vi "Glove box startup.vi"() -> ()   [LabVIEW 2017]
uses:
  <instrlib>/SST sensing O2 sensor/SST sensing O2 sensor.lvlib
panel:
  out "O2 free reached":bool
  in  "Off threshold %":dbl=1.0
  out "O2 level %":dbl
  out "O2 level Chart":dbl(graph)
  in  "Start N2 purge":bool
  in  "stop":bool
  out "Sensor status":string="Idle"
  in  "O2 sensor On/Off":bool
  in  "O2 sensor COM":refnum<visa-resource-name>="COM18"
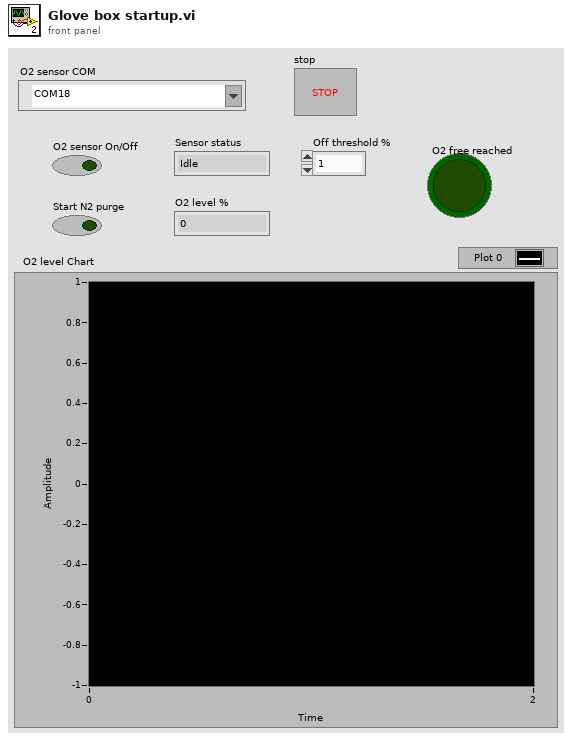
[diagram p1: front panel]
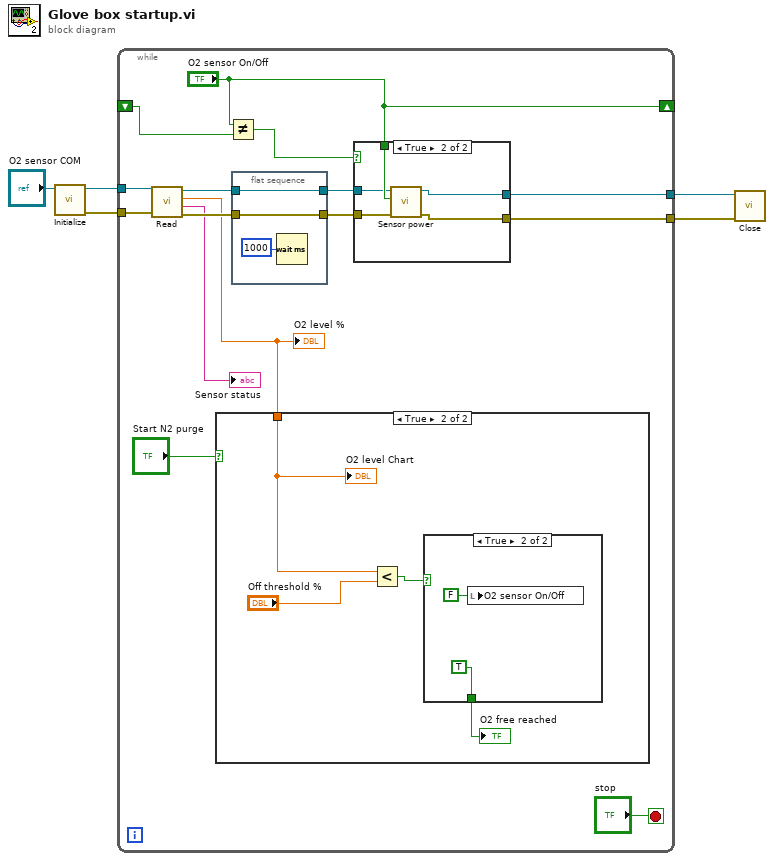
[diagram p0: block diagram]
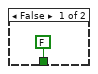
[diagram p3: hidden frame]
diagram:
  n1 = call <instrlib>:"Initialize.vi"("COM port"="O2 sensor COM") -> ("error out"=w3:errorcluster, "Modbus instance"=w4:refnum<class "Modbus Master.lvclass">)  [unwired: 9 in]
  n2 = while {
    tunnel: w4 -> [w20]
    tunnel: w3 -> [w19]
    shift-right: ["O2 sensor On/Off"] -> _
    shift-left: _ -> [w17]
    tunnel: [w10] -> w2
    tunnel: [w9] -> w1
    stop <- "stop" stop-if-true
    n3 = call <instrlib>:"Read.vi"("error in (no error)"=w19, "Modbus master in"=w20) -> ("error out"=w12:errorcluster, "Status"=→"Sensor status":string, "O2 level %"=w6:dbl, "Modbus master out"=w14:refnum<class "Modbus Master.lvclass">)  [unwired: 6 in]
    "O2 level %" <- w6
    n4 = case shown="True" "Start N2 purge" {
      tunnel: w6 -> [_ w24]
      frame False {
      }
      frame True {
        n5 = Less?(x=w24, y="Off threshold %") -> (x < y?=w22:bool)
        n6 = case shown="True" w22 {
          tunnel: [FALSE ("O2 free reached") TRUE ("O2 free reached")] -> w21
          frame False {
          }
          frame True {
            n7 = local write "O2 sensor On/Off"(FALSE ("O2 sensor On/Off")) -> ()
          }
        }
        "O2 free reached" <- w21
        "O2 level Chart" <- w24
      }
    }
    n8 = Not Equal?(x="O2 sensor On/Off", y=w17) -> (x != y?=w16:bool)
    n9 = flat-sequence {
      tunnel: [w30] -> w15
      tunnel: w14 -> [w30]
      tunnel: [w29] -> w13
      tunnel: w12 -> [w29]
      frame #0 {
        n10 = Wait (ms)(milliseconds to wait=u32 1000) -> ()  [unwired: 1 out]
      }
    }
    n11 = case shown="True" w16 {
      tunnel: "O2 sensor On/Off" -> [_ w37]
      tunnel: w15 -> [w32 w36]
      tunnel: w13 -> [w31 w35]
      tunnel: [w32 w34] -> w10
      tunnel: [w31 w33] -> w9
      frame False {
      }
      frame True {
        n12 = call <instrlib>:"Sensor power.vi"("error in (no error)"=w35, "On/Off"=w37, "Modbus master in"=w36) -> ("error out"=w33:errorcluster, "Modbus master out"=w34:refnum<class "Modbus Master.lvclass">)  [unwired: 7 in]
      }
    }
  }
  n13 = call <instrlib>:"Close.vi"("error in (no error)"=w1, "Modbus master in"=w2) -> ()  [unwired: 9 in, 1 out]
